vi "Shooter Speeds.vi"(6 "Right Bumper":bool, 9 "Robot Angle":T1, 10 "Shooter Angle":T1, 11 "Shooter Speeds":dbl[](array[numeric])) -> (3 "f":dbl)   [LabVIEW 2012]
uses:
  <vilib>/Rock Robotics/WPI/Solenoid/WPI_SolenoidValue.ctl
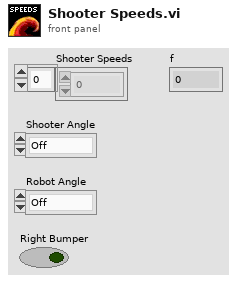
[diagram p1: front panel]
types:
  T1 = typedef "WPI_SolenoidValue.ctl" = enum16{"Off", "On", "Forward", "Reverse"}
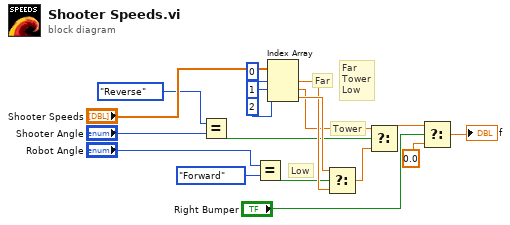
[diagram p0: block diagram]
diagram:
  # "Far\nTower\nLow"
  # "Low"
  # "Tower"
  # "Far"
  n1 = Equal?(x=WPI_SolenoidValue."Reverse" ("Solenoids.Robot Angle"), y="Shooter Angle") -> (x = y?=w2:bool)
  n2 = Equal?(x="Robot Angle", y=WPI_SolenoidValue."Forward" ("Solenoids.Robot Angle")) -> (x = y?=w4:bool)
  n3 = Index Array(array="Shooter Speeds", index #1=0 ("index"), index #2=1 ("index"), index #3=2 ("index")) -> (element #1=w16:dbl, element #2=w14:dbl, element #3=w17:dbl)
  n4 = Select(t=w17, s=w4, f=w16) -> (s? t:f=w3:dbl)
  n5 = Select(t=w14, s=w2, f=w3) -> (s? t:f=w6:dbl)
  n6 = Select(t=w6, s="Right Bumper", f=0.0) -> (s? t:f=→"f":dbl)
